vi "Builder.Wait for Command.vi"(8 "error in (no error)":errorcluster, 11 "Builder in":refnum<class "Builder.lvclass">) -> (0 "error out":errorcluster, 1 "command action":T1, 2 "command data":T2, 3 "Builder out":refnum<class "Builder.lvclass">)   [LabVIEW 2016, in "DSF.Engine.lvlib" / "Builder.lvclass"]
uses:
  Builder.lvclass
  Interface/DSF.Engine.Interface.Builder.Command Data.ctl
  Interface/DSF.Engine.Interface.Builder.Command.ctl
  Builder.lvclass/Builder.ctl
  Interface/DSF.Engine.Interface.Builder.Read.Command.vi
  Interface/DSF.Engine.Interface.Builder.lvclass
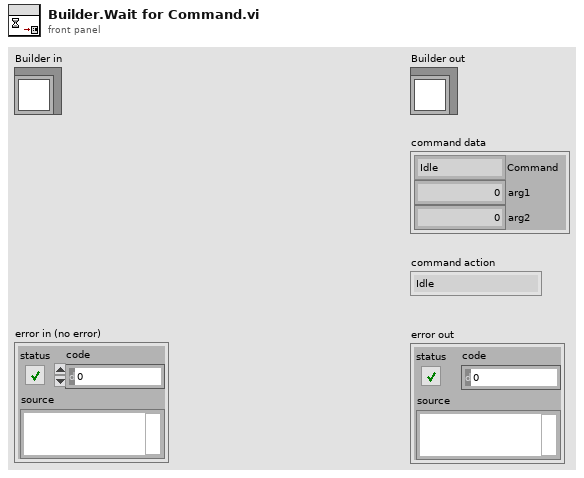
[diagram p1: front panel]
types:
  T1 = typedef "DSF.Engine.lvlib/DSF.Engine.Interface.Builder.lvclass/DSF.Engine.Interface.Builder.Command.ctl" = enum8{"Idle", "Initialize", "Build Buffer", "Parse Buffer", "Shutdown"}
  T2 = typedef "DSF.Engine.lvlib/DSF.Engine.Interface.Builder.lvclass/DSF.Engine.Interface.Builder.Command Data.ctl" = cluster{"Command":T1, "arg1":u64, "arg2":u64}
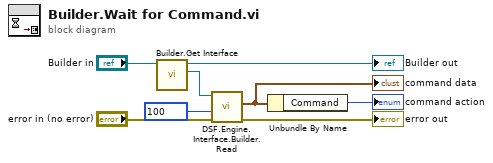
[diagram p0: block diagram]
diagram:
  n1 = call "Builder.Get Interface.vi"("Builder in"="Builder in") -> ("Builder Interface"=w3:refnum<class "DSF.Engine.Interface.Builder.lvclass">, "Builder out"=→"Builder out":refnum<class "Builder.lvclass">)  [unwired: 9 in]
  n2 = call-poly "DSF.Engine.Interface.Builder.Read.vi"("error in (no error)"="error in (no error)", "timeout in ms (0)"=100, "Builder Interface in"=w3) -> ("error out"=→"error out":errorcluster, "command"=w2:T2)  [unwired: 4 in, 3 out]
  "command data" <- w2
  n3 = Unbundle By Name(w2) -> ("Command"=→"command action":T1)
